vi "Direct.vi"(7 "Consulter Bilan":bool) -> (1 "Date":string, 2 "Image":T2(plugin-control), 3 "Localisation":string, 5 "Nombre de \nvéhicules suspects:":dbl, 6 "Nombre de véhicules:":dbl)   [LabVIEW 2024]
uses:
  <vilib>/Utility/miscctls.llb/LVPoint32TypeDef.ctl
  Assets/text_indicator.ctl
panel:
  in  "File Path 2":path
  in  "Image Name 2":string="untitled"
  in  "File Path":path
  in  "Image Name":string="untitled"
  in  "Coords 2":T1={"Horizontal"=20, "Vertical"=20}
  in  "Coords":T1={"Horizontal"=60, "Vertical"=60}
  in  "stop":bool
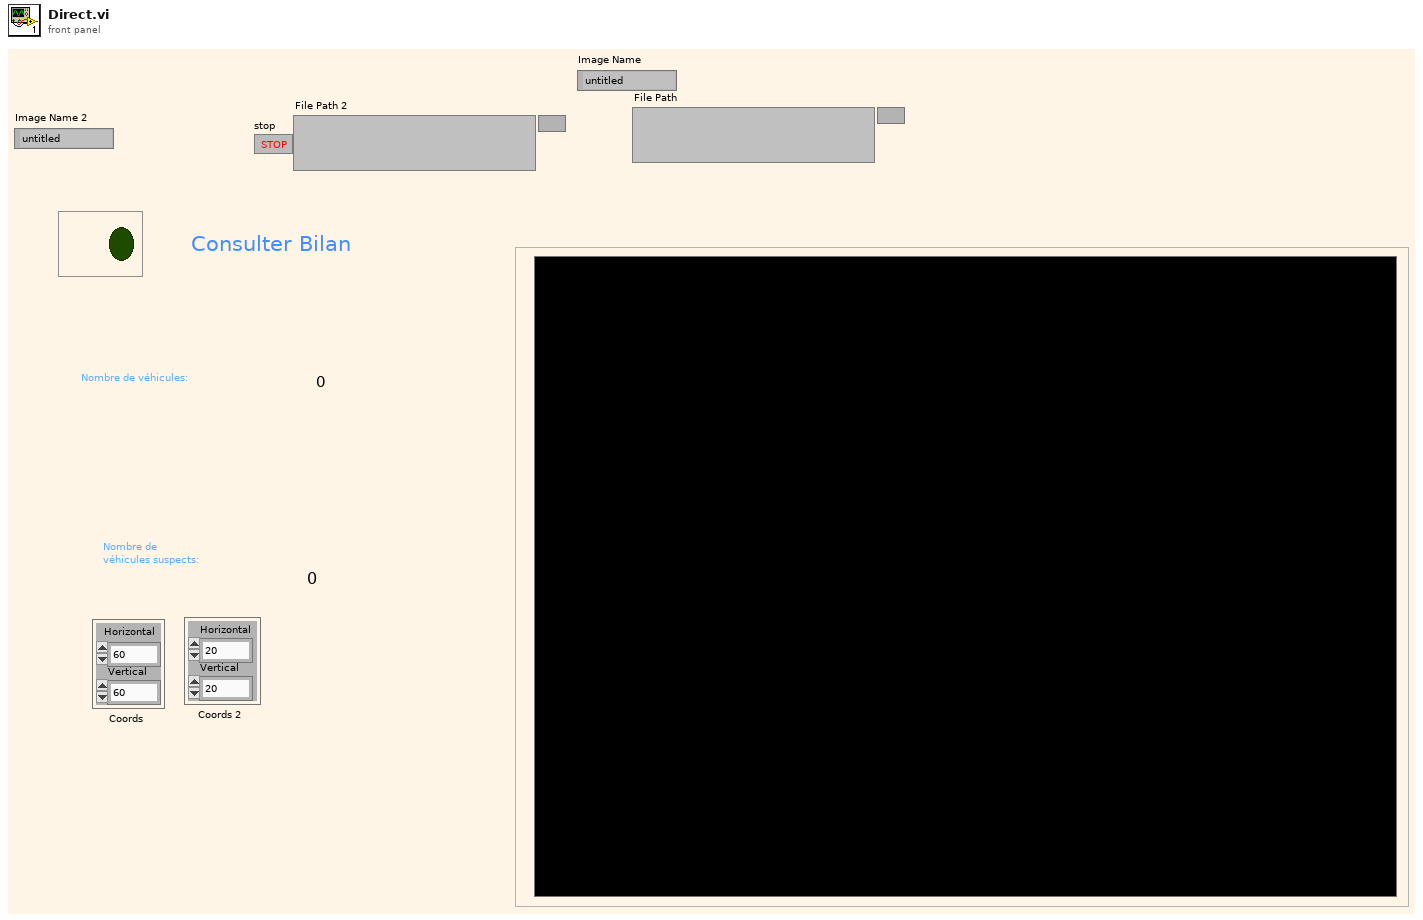
[diagram p1: front panel]
types:
  T1 = typedef "LVPoint32TypeDef.ctl" = cluster{"Horizontal":i32, "Vertical":i32}
  T2 = typedef "IMAQ Image.ctl" = refnum<image>
  T3 = typedef "Image Type" = u32
  T4 = cluster{"Horizontal":i32, "Vertical":i32, "Horizontal":i32, "Vertical":i32}
  T5 = typedef "text_indicator.ctl" = string
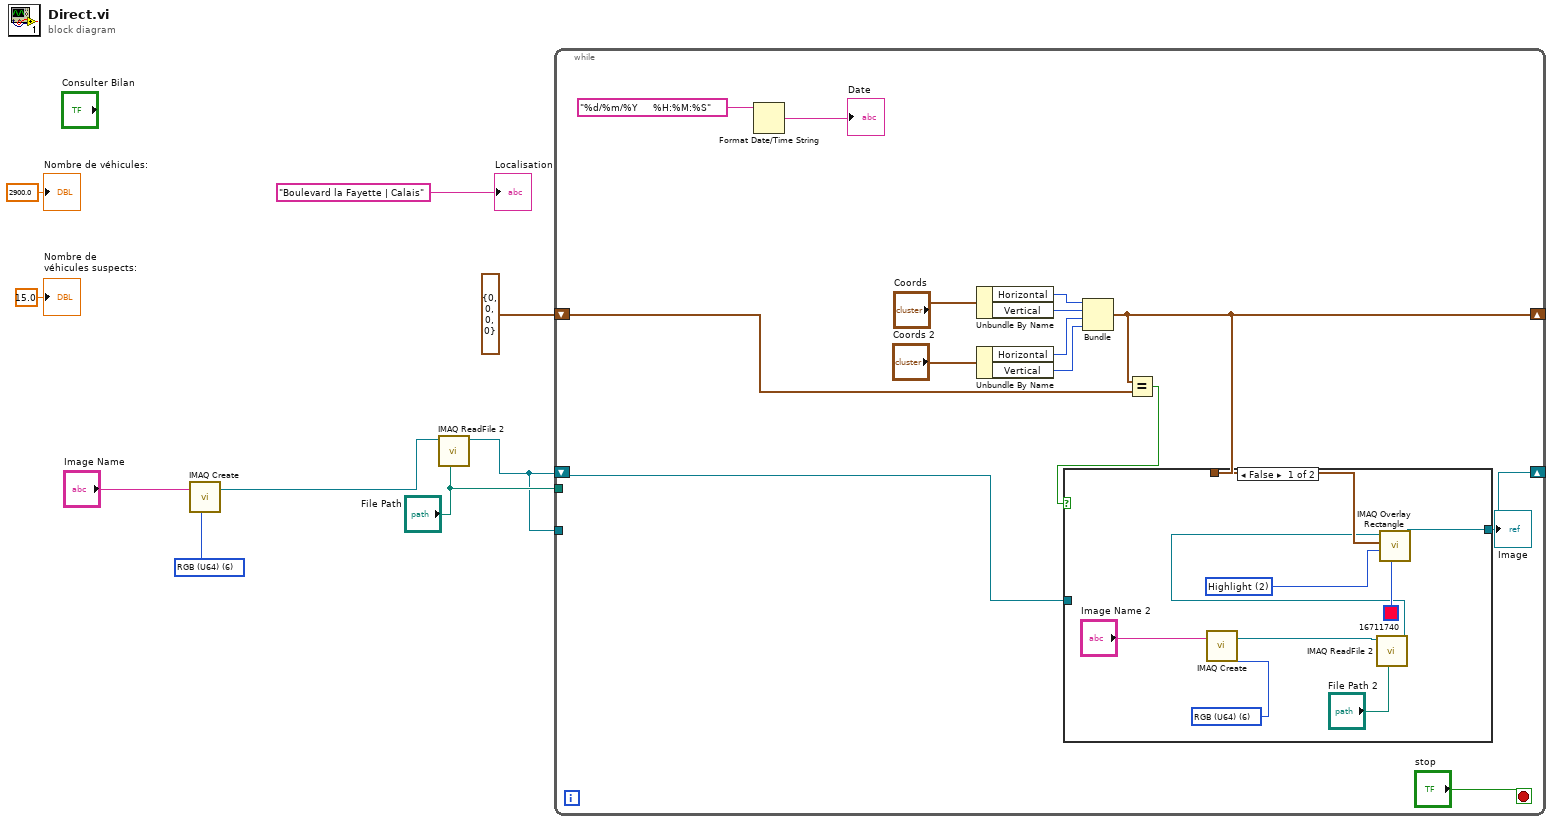
[diagram p0: block diagram]
diagram:
  w4 = T3 6 items=["Grayscale (U8)", "Grayscale (I16)", "Grayscale (SGL)", "Complex (CSG)", "RGB (U32)", "HSL (U32)", "RGB (U64)", "Grayscale (U16)"] ("Image Type")
  n1 = call "IMAQ Create"("Image Name"="Image Name", "Image Type"=w4) -> ("New Image"=w2:T2)  [unwired: 3 in, 1 out]
  n2 = call "IMAQ ReadFile 2"("File Path"="File Path", "Image"=w2) -> ("Image Out"=w1:T2)  [unwired: 5 in, 4 out]
  n3 = while {
    shift-right: [w15] -> _
    shift-left: T4 {"Horizontal"=0, "Vertical"=0, "Horizontal"=0, "Vertical"=0} -> [w12]
    shift-right: [w11] -> _
    shift-left: w1 -> [w10]
    tunnel: "File Path" -> [_]
    tunnel: w1 -> [_]
    stop <- "stop" stop-if-true
    n4 = Format Date/Time String(time format string (%c)="%d/%m/%Y     %H:%M:%S") -> (date/time string=→"Date":string)  [unwired: 2 in]
    n5 = Unbundle By Name("Coords") -> ("Horizontal"=w23:i32, "Vertical"=w22:i32)
    n6 = Unbundle By Name("Coords 2") -> ("Horizontal"=w21:i32, "Vertical"=w20:i32)
    n7 = Bundle("Horizontal"=w23, "Vertical"=w22, "Horizontal"=w21, "Vertical"=w20) -> (w15:T4)  [unwired: 1 in]
    n8 = Equal?(x=w15, y=w12) -> (x = y?=w16:bool)
    n9 = case shown="False" w16 {
      tunnel: [w30 w33] -> w11
      tunnel: w15 -> [w29 _]
      tunnel: w10 -> [_ w33]
      frame False {
        w25 = T3 6 items=["Grayscale (U8)", "Grayscale (I16)", "Grayscale (SGL)", "Complex (CSG)", "RGB (U32)", "HSL (U32)", "RGB (U64)", "Grayscale (U16)"] ("Image Type")
        w31 = u32 2 items=["Frame", "Fill", "Highlight"] ("Drawing Mode (Frame)")
        n10 = call "IMAQ Create"("Image Name"="Image Name 2", "Image Type"=w25) -> ("New Image"=w28:T2)  [unwired: 3 in, 1 out]
        n11 = call "IMAQ ReadFile 2"("File Path"="File Path 2", "Image"=w28) -> ("Image Out"=w24:T2)  [unwired: 5 in, 4 out]
        n12 = call "IMAQ Overlay Rectangle"("Color"=u32 16711740, "Drawing Mode (Frame)"=w31, "Rectangle"=w29, "Image"=w24) -> ("Image Out"=w30:T2)  [unwired: 6 in, 1 out]
      }
      frame True {
      }
    }
    "Image" <- w11
  }
  "Nombre de véhicules:" <- 2900.0 ("Nombre de véhicules:")
  "Nombre de \nvéhicules suspects:" <- 15.0 ("Nombre de \nvéhicules suspects:")
  "Localisation" <- T5 "Boulevard la Fayette | Calais" ("Localisation")
